vi "Execute with Default Process Model.vi"() -> ()   [LabVIEW 2020]
uses:
  Execution Options.ctl
  Set Entry Sequence.vi
  Set Sequence File.vi
  Get Result Status.vi
  Engine/Engine.lvclass
  Execution.lvclass
panel:
  in  "Entry Point":string="Single Pass"
  out "Status":string
  in  "SequenceFile Path":path=path "C:/Users/Public/Documents/National Instruments/TestStand 2019 (32-bit)/Examples/Demos/Computer Motherboard Test/LabVIEW/Computer Motherboard Test Sequence.seq"
  # "1."
  # "2."
  # "1. Select the sequence file you'd like to run.\n\n2. Enter the name of the entry point to use in the process model. This is usually 'Test UUTs' or 'Single Pass' for models that ship with TestStand."
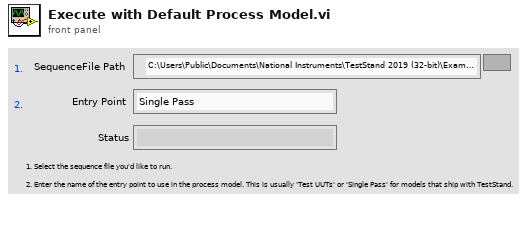
[diagram p1: front panel]
types:
  T1 = typedef "TSS.lvlib/Execution.lvclass/Execution Options.ctl" = cluster{"Use Default Model":bool, "Release Related Sessions":bool}
  T2 = typedef "TSS.lvlib/Engine.lvclass/Session Handle.ctl" = refnum<data-value>
  T3 = typedef "TSS.lvlib/SequenceFile.lvclass/Session Handle.ctl" = refnum<data-value>
  T4 = typedef "TSS.lvlib/Execution.lvclass/Session Handle.ctl" = refnum<data-value>
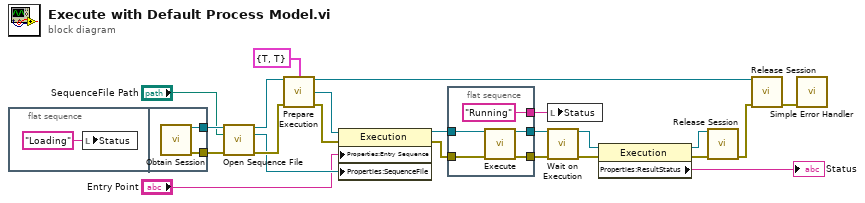
[diagram p0: block diagram]
diagram:
  n1 = flat-sequence {
    tunnel: [w26] -> w23
    tunnel: [w25] -> w17
    frame #0 {
      n2 = local write "Status"("Loading" ("Status")) -> ()
    }
    frame #1 {
      n3 = call "Obtain Session.vi"() -> ("Session Handle"=w26:T2, "error out"=w25:errorcluster)  [unwired: 14 in]
    }
  }
  n4 = call "Open Sequence File.vi"("Engine in"=w23, "File Path"="SequenceFile Path", "error in (no error)"=w17) -> ("Session Handle out"=w7:T2, "SequenceFile"=w5:T3, "error out"=w6:errorcluster)  [unwired: 10 in]
  n5 = call "Prepare Execution.vi"("Session Handle in"=w7, "Options (Default)"=T1 {"Use Default Model"=TRUE, "Release Related Sessions"=TRUE}, "error in (no error)"=w6) -> ("Session Handle out"=w14:T2, "Execution"=w22:T4, "error out"=w16:errorcluster)  [unwired: 10 in]
  n6 = property class="Execution"(reference=w22, error in=w16, "Properties:Entry Sequence"="Entry Point", "Properties:SequenceFile"=w5) -> (reference out=w21:T4, error out=w18:errorcluster)
  n7 = flat-sequence {
    tunnel: w21 -> [w31]
    tunnel: [w30] -> w20
    tunnel: [w29] -> w19
    tunnel: w18 -> [w28]
    tunnel: ["Running" ("Status")] -> w3
    frame #0 {
      n8 = call "Execute.vi"("Session Handle in"=w31, "error in (no error)"=w28) -> ("Session Handle out"=w30:T4, "error out"=w29:errorcluster)  [unwired: 12 in]
    }
  }
  n9 = local write "Status"(w3) -> ()
  n10 = call "Wait on Execution.vi"("Session Handle in"=w20, "error in (no error)"=w19) -> ("Session Handle out"=w13:T4, "error out"=w12:errorcluster)  [unwired: 11 in, 1 out]
  n11 = property class="Execution"(reference=w13, error in=w12) -> (reference out=w10:T4, error out=w11:errorcluster, "Properties:ResultStatus"=→"Status":string)
  n12 = call "Release Session.vi"("Session Handle"=w10, "error in (no error)"=w11) -> ("error out"=w15:errorcluster)  [unwired: 13 in]
  n13 = call "Release Session.vi"("Session Handle"=w14, "error in (no error)"=w15) -> ("error out"=w8:errorcluster)  [unwired: 13 in]
  n14 = call <vilib>:"Simple Error Handler.vi"("error in (no error)"=w8) -> ()  [unwired: 4 in, 5 out]
